vi "Send move to stages.vi"(8 "error in (no error)":errorcluster, 11 "Tomo in":refnum<class "Tomo.lvclass">) -> (0 "error out":errorcluster, 3 "Tomo out":refnum<class "Tomo.lvclass">)   [LabVIEW 2012, in "Tomo.lvclass"]
uses:
  Tomo.lvclass
  <vilib>/Distrio/Murmex/GenericMessage/GenericMessage.lvclass
  <vilib>/Distrio/Murmex/Message/Message.lvclass
  <vilib>/Distrio/Murmex/Murmex/Murmex.lvclass
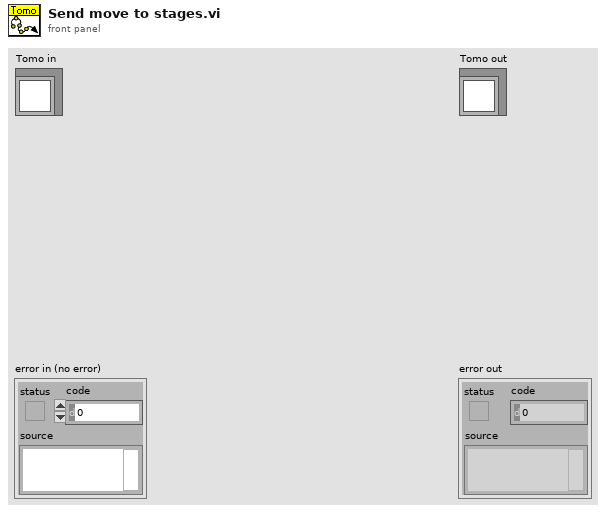
[diagram p1: front panel]
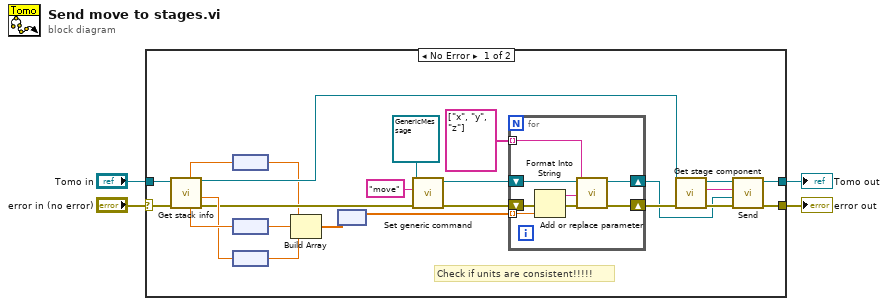
[diagram p0: block diagram]
diagram:
  n1 = case shown="No Error" "error in (no error)" {
    selector: "error in (no error)" -> [w25 w38]
    tunnel: [w15 w38] -> w3
    tunnel: [w16 w37] -> w1
    tunnel: "Tomo in" -> [w26 w37]
    frame No Error {
      # "Check if units are consistent!!!!!"
      n2 = call-dynamic "Get stack info.vi"("error in (no error)"=w25, "Tomo in"=w26) -> ("error out"=w9:errorcluster, "Z start"=w22:dbl, "Tomo out"=w8:refnum<class "Tomo.lvclass">, "Y position"=w23:dbl, "X position"=w24:dbl)  [unwired: 4 in, 1 out]
      n3 = node(w24) -> (w5:dbl[unit])
      n4 = node(w23) -> (w7:dbl[unit])
      n5 = node(w22) -> (w6:dbl[unit])
      n6 = Build Array(w5, w7, w6) -> (w18:dbl[unit][])
      n7 = node(w18) -> (w10:dbl[])
      n8 = call <vilib>:"Set generic command.vi"("error in (no error)"=w9, "generic command"="move" ("command string"), "GenericMessage in"=refnum<class "GenericMessage.lvclass"> refnum ("Murmex.lvlib:GenericMessage")) -> ("error out"=w21:errorcluster, "GenericMessage out"=w20:refnum<class "GenericMessage.lvclass">)  [unwired: 7 in]
      n9 = for {
        shift-right: [w30] -> w14
        shift-left: w21 -> [w36]
        shift-right: [w31] -> w11
        shift-left: w20 -> [w35]
        tunnel: string[] ["x", "y", "z"] -> [w33] mode=indexing
        tunnel: w10 -> [w32] mode=indexing
        n10 = Format Into String(error in=w36, w32) -> (resulting string=w29:string, error out=w34:errorcluster)  [unwired: 2 in]
        n11 = call <vilib>:"Add or replace parameter.vi"("error in (no error)"=w34, "value"=w29, "name"=w33, "Message in"=w35) -> ("error out"=w30:errorcluster, "Message out"=w31:refnum<class "GenericMessage.lvclass">)  [unwired: 6 in]
      }
      n12 = call-dynamic "Get stage component.vi"("error in (no error)"=w14, "Tomo in"=w8) -> ("error out"=w13:errorcluster, "stage component"=w12:string, "Tomo out"=w17:refnum<class "Tomo.lvclass">)  [unwired: 7 in]
      n13 = call <vilib>:"Send.vi"("error in (no error)"=w13, "Message"=w11, "recipient"=w12, "Murmex in"=w17) -> ("error out"=w15:errorcluster, "Murmex out"=w16:refnum<class "Tomo.lvclass">)  [unwired: 6 in]
    }
    frame Error {
    }
  }
  "error out" <- w3
  "Tomo out" <- w1
